vi "Group Already Exists.vi"(7 "caller name":string, 8 "error in (no error)":errorcluster, 10 "found?":bool, 11 "Group":string) -> (0 "error out":errorcluster)   [LabVIEW 2020, in "Current Value Table(Rebuild).lvlib"]
doc: "This VI throws an error if a selected group could not be found in the calling VI."
uses:
  Current Value Table(Rebuild).lvlib
panel:
  # "This should append the error onto the source, (ie provide a list of items not found)."
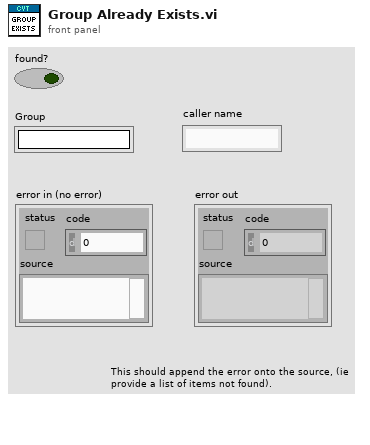
[diagram p1: front panel]
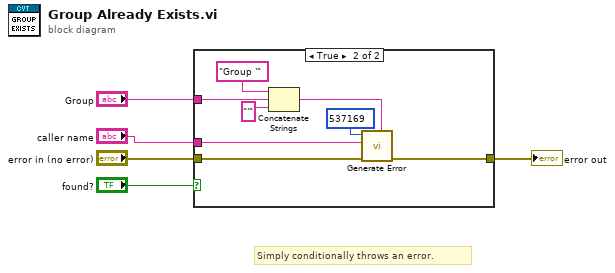
[diagram p0: block diagram]
diagram:
  # "Simply conditionally throws an error."
  n1 = case shown="True" "found?" {
    tunnel: "error in (no error)" -> [w6 w10]
    tunnel: [w6 w9] -> w4
    tunnel: "Group" -> [_ w14]
    tunnel: "caller name" -> [_ w7]
    frame False {
    }
    frame True {
      n2 = Concatenate Strings("Group '" ("string"), w14, "'" ("string")) -> (w8:string)
      n3 = call "Generate Error.vi"("<append> (\"\")"=w8, "error in"=w10, "caller name"=w7, "code"=537169) -> ("error out"=w9:errorcluster)  [unwired: 7 in]
    }
  }
  "error out" <- w4
